vi "FilterVoltammetryData.vi"(8 "error in (no error)":errorcluster, 11 "Input":dbl[](array[numeric])) -> (0 "error out":errorcluster, 3 "Output":dbl[](array[numeric]))   [LabVIEW 2015, in "ReDeX.lvlib"]
uses:
  ReDeX.lvlib
  C:/ReDeX/ReDeX.dll
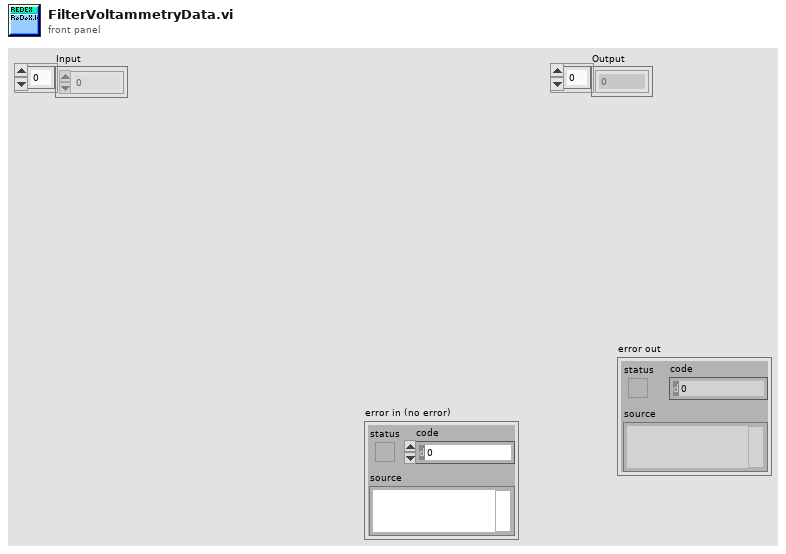
[diagram p1: front panel]
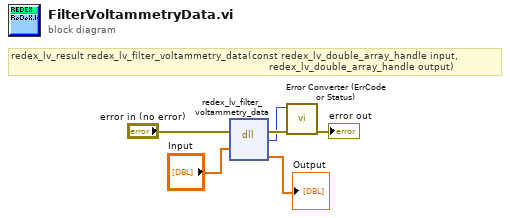
[diagram p0: block diagram]
diagram:
  # "redex_lv_result redex_lv_filter_voltammetry_data(const redex_lv_double_array_handle input,\n                                                                                      redex_lv_double_array_handle output)"
  n1 = dll-call lib="C:/ReDeX/ReDeX.dll" fn="redex_lv_filter_voltammetry_data"(error in="error in (no error)", "input"="Input") -> (error out=w5:errorcluster, "return type"=w4:u32, "output"=→"Output":dbl[])  [unwired: 4 in, 1 out]
  n2 = call "Error Converter (ErrCode or Status).vi"("error in (no error)"=w5, "error code"=w4) -> ("error out"=→"error out":errorcluster)  [unwired: 9 in]
